vi "32xx_Cde _U_I.vi"(8 "error in (no error)":errorcluster, 9 "Valeur (V/A)":dbl=2.5 format="%.2g", 10 "Select Voie":i32(ring)=3 items=["CH 1"=1, "CH 2"=2, "CH 3"=3], 11 "VISA resource name":refnum<visa-resource-name>="COM3") -> (0 "error out":errorcluster, 3 "VISA resource name out":refnum<visa-resource-name>="COM3")   [LabVIEW 2020]
doc: "This elementary program is used to write a voltage or current setpoint, to choose the channel (ALR3206 D & T).\n\nCe programme élémentaire permet d'écrire une consigne de tension ou de courant, \nde choisir la voie (ALR3206 D & T)."
panel:
  in  "ON/OFF":T1=1 items=["OFF", "ON"]
  in  "Local/Remote":enum16{"Local", "Remote"}(ring)=enum."Remote"
  in  "Produit":T2(ring)
  in  "Chaîne\nSelect.\nParam.":string(combo)="VOLT" caption="Select. Param."
  # "© 2020 elc ALL RIGHTS RESERVED"
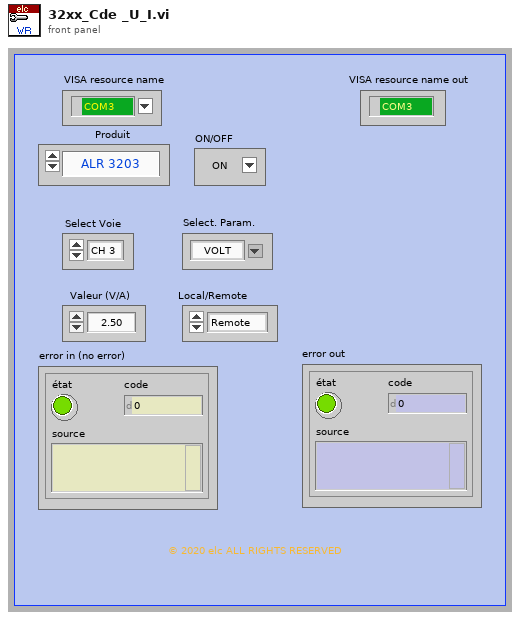
[diagram p1: front panel]
types:
  T1 = typedef "32xx_MenuDeroulant_ON_OFF.ctl" = u16
  T2 = enum16{"ALR 3203", "ALR 3220", "ALR 3206D", "ALR 3206T"}
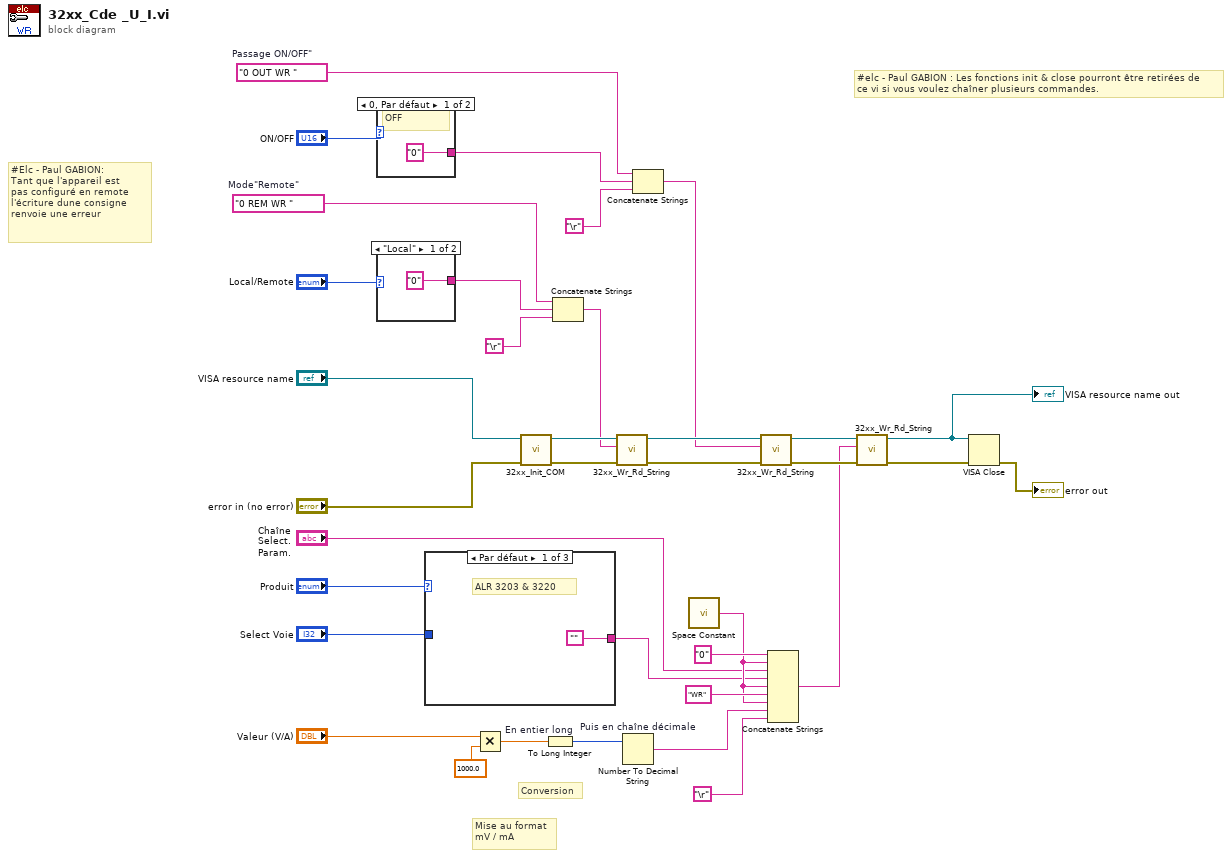
[diagram p0: block diagram]
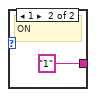
[diagram p2: hidden frame]
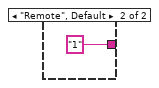
[diagram p3: hidden frame]
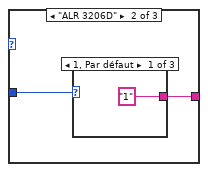
[diagram p4: hidden frame]
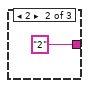
[diagram p5: hidden frame]
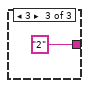
[diagram p6: hidden frame]
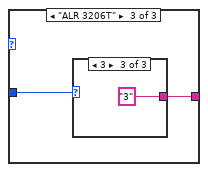
[diagram p7: hidden frame]
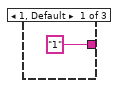
[diagram p8: hidden frame]
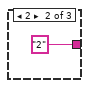
[diagram p9: hidden frame]
diagram:
  w34 = "0 OUT WR "  # Passage ON/OFF"
  w7 = "0 REM WR "  # Mode"Remote"
  # "#Elc - Paul GABION:\nTant que l'appareil est\npas configuré en remote\nl'écriture dune consigne \nrenvoie une erreur"
  # "Mise au format\nmV / mA"
  # "Conversion"
  # "#elc - Paul GABION : Les fonctions init & close pourront être retirées de\nce vi si vous voulez chaîner plusieurs commandes."
  n1 = case shown="0, Par défaut" "ON/OFF" {
    tunnel: ["0" ("chaîne") "1" ("chaîne")] -> w1
    frame 0, Default {
      # "OFF"
    }
    frame 1 {
      # "ON"
    }
  }
  n2 = case shown="\"Local\"" "Local/Remote" {
    tunnel: ["0" ("chaîne") "1" ("chaîne")] -> w6
    frame "Local" {
    }
    frame "Remote", Default {
    }
  }
  n3 = case shown="Par défaut" "Produit" {
    tunnel: "Select Voie" -> [_ w42 w47]
    tunnel: ["" w41 w46] -> w12
    frame Default {
      # "ALR 3203 & 3220"
    }
    frame "ALR 3206D" {
      n4 = case shown="1, Par défaut" w42 {
        tunnel: ["1" ("chaîne") "2" ("chaîne") "2" ("chaîne")] -> w41
        frame 1, Default {
        }
        frame 2 {
        }
        frame 3 {
        }
      }
    }
    frame "ALR 3206T" {
      n5 = case shown="3" w47 {
        tunnel: ["1" ("chaîne") "2" ("chaîne") "3" ("chaîne")] -> w46
        frame 1, Default {
        }
        frame 2 {
        }
        frame 3 {
        }
      }
    }
  }
  n6 = Multiply(x="Valeur (V/A)", y=1000.0) -> (x*y=w15:dbl)
  n7 = call "32xx_Init_COM.vi"("Entrée d'erreur"="error in (no error)", "Port d'entrée"="VISA resource name") -> ("Sortie d'erreur"=w29:errorcluster, "Port de sortie"=w30:refnum<visa-resource-name>)  [unwired: 7 in, 1 out]
  n8 = To Long Integer "En entier long"(number=w15) -> (32bit integer=w20:i32)
  n9 = Concatenate Strings(w7, w6, "\r") -> (w3:string)
  n10 = call "32xx_Wr_Rd_String.vi"("entrée d'erreur"=w29, "String In"=w3, "Visa In"=w30) -> ("sortie d'erreur"=w27:errorcluster, "Visa Out"=w28:refnum<visa-resource-name>)  [unwired: 4 in, 3 out]
  n11 = Number To Decimal String "Puis en chaîne décimale"(number=w20) -> (decimal integer string=w14:string)  [unwired: 1 in]
  n12 = Concatenate Strings(w34, w1, "\r") -> (w26:string)
  n13 = call <vilib>:"Space Constant.vi"() -> ("String"=w16:string)
  n14 = call "32xx_Wr_Rd_String.vi"("entrée d'erreur"=w27, "String In"=w26, "Visa In"=w28) -> ("sortie d'erreur"=w24:errorcluster, "Visa Out"=w25:refnum<visa-resource-name>)  [unwired: 4 in, 3 out]
  n15 = Concatenate Strings("0" ("chaîne"), w16, "Chaîne\nSelect.\nParam.", w12, w16, "WR" ("chaîne"), w16, w14, "\r") -> (w9:string)
  n16 = call "32xx_Wr_Rd_String.vi"("entrée d'erreur"=w24, "String In"=w9, "Visa In"=w25) -> ("sortie d'erreur"=w22:errorcluster, "Visa Out"=w23:refnum<visa-resource-name>)  [unwired: 4 in, 3 out]
  "VISA resource name out" <- w23
  n17 = VISA Close(VISA resource name=w23, error in (no error)=w22) -> (error out=→"error out":errorcluster)
